vi "Complex Outer Product.vi"(2 "Y Vector":cdb[](array[numeric]) format="%.2f", 3 "X Vector":cdb[](array[numeric]) format="%.2f") -> (0 "error":i32, 1 "Outer Product":T1)   [LabVIEW 2020, in "NI_AALBase.lvlib"]
doc: "Computes the outer product of <B>X Vector</B> and <B>Y Vector</B>. The data types you wire to the <B>X Vector</B> and <B>Y Vector</B> inputs determine the polymorphic instance to use."
uses:
  NI_AALBase.lvlib
  ComplexMatrix.ctl
  <resource>/lvanlys.dll
  NI_Matrix.lvlib
panel:
  # "Complex Outer Product"
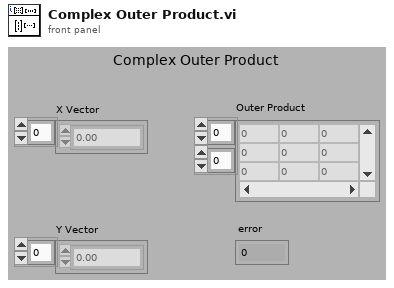
[diagram p1: front panel]
types:
  T1 = typedef "NI_Matrix.lvlib/ComplexMatrix.ctl" = cdb[][]
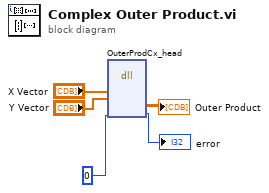
[diagram p0: block diagram]
diagram:
  n1 = dll-call lib="C:/Program Files (x86)/National Instruments/LabVIEW 2020/resource/lvanlys.*" fn="OuterProdCx_head"("X Vector"="X Vector", "Y Vector"="Y Vector", 0) -> ("Outer Product"=→"Outer Product":T1, →"error":i32)  [unwired: 7 in, 2 out]
